vi "Connect Pane.vi"(0 "connect pane":refnum<vi>, 1 "Controls[]":refnum<vi>[](array[refnum]), 11 "error in":errorcluster {"code" format="%.0x"}) -> (3 "Controls[] output":refnum<vi>[](array[refnum]), 4 "connect pane out":refnum<vi>, 15 "error out":errorcluster {"code" format="%.0x"})   [LabVIEW 2018, in "NISAST VI Scripting.lvlib" / "VI.lvlib" / "Connector.lvlib"]
uses:
  Connector.lvlib
  Front Panel/Front Panel.lvlib
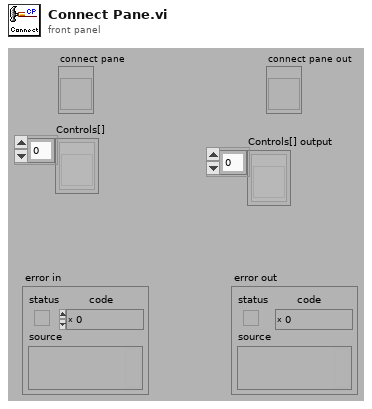
[diagram p1: front panel]
types:
  T1 = typedef "NISAST VI Scripting.lvlib/VI.lvlib/Front Panel.lvlib/Connector Pane Type.ctl" = enum16{"4-2-2-4", "5-2-2-2-5", "Others"}
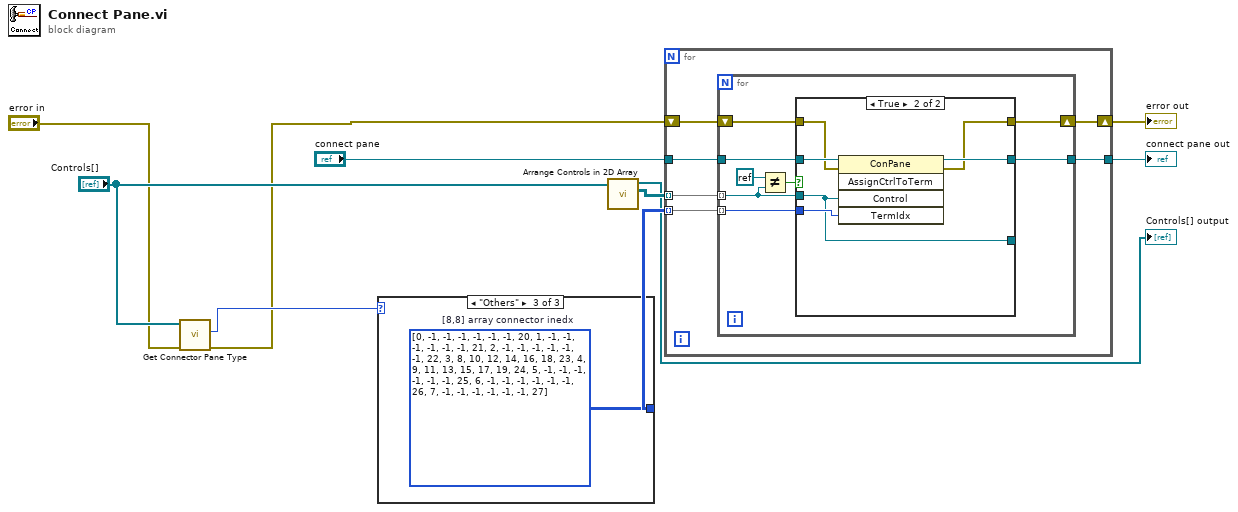
[diagram p0: block diagram]
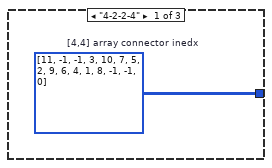
[diagram p2: hidden frame]
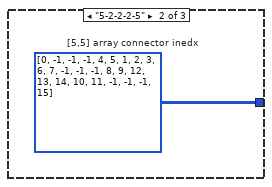
[diagram p3: hidden frame]
diagram:
  n1 = call "Get Connector Pane Type.vi"("error in (no error)"="error in", "Controls[]"="Controls[]") -> ("error out"=w1:errorcluster, "Connector Pane Type"=w3:T1)  [unwired: 7 out]
  n2 = case shown="\"Others\"" w3 {
    tunnel: [w11 w12 w13] -> w6
    frame "4-2-2-4" {
      w11 = i32[][] [[11, -1, -1, 3], [10, 7, 5, 2], [9, 6, 4, 1], [8, -1, -1, 0]]  # [4,4] array connector inedx
    }
    frame "5-2-2-2-5" {
      w12 = i32[][] [[0, -1, -1, -1, 4], [5, 1, 2, 3, 6], [7, -1, -1, -1, 8], [9, 12, 13, 14, 10], [11, -1, -1, -1, 15]]  # [5,5] array connector inedx
    }
    frame "Others" {
      w13 = i32[][] [[0, -1, -1, -1, -1, -1, -1, 20], [1, -1, -1, -1, -1, -1, -1, 21], [2, -1, -1, -1, -1, -1, -1, 22], [3, 8, 10, 12, 14, 16, 18, 23], [4, 9, 11, 13, 15, 17, 19, 24], [5, -1, -1, -1, -1, -1, -1, 25], [6, -1, -1, -1, -1, -1, -1, 26], [7, -1, -1, -1, -1, -1, -1, 27]]  # [8,8] array connector inedx
    }
  }
  n3 = call "Arrange Controls in 2D Array.vi"("Controls[]"="Controls[]") -> ("controls 2D[]"=w7:refnum<vi>[][], "Controls[]"=→"Controls[] output":refnum<vi>[])  [unwired: 1 in, 8 out]
  n4 = for {
    tunnel: w7 -> [w19] mode=indexing
    tunnel: w6 -> [w18] mode=indexing
    tunnel: "connect pane" -> [w17]
    shift-right: [w15] -> w8
    shift-left: w1 -> [w16]
    tunnel: [w14] -> w9
    n5 = for {
      tunnel: w19 -> [w24] mode=indexing
      tunnel: w18 -> [w26] mode=indexing
      tunnel: w17 -> [w25]
      shift-right: [w21] -> w15
      shift-left: w16 -> [w22]
      tunnel: [w20] -> w14
      n6 = Not Equal?(x=refnum<k0> refnum, y=w24) -> (x != y?=w27:bool)
      n7 = case shown="True" w27 {
        tunnel: w24 -> [w28 w32]
        tunnel: w26 -> [_ w34]
        tunnel: w25 -> [w29 w36]
        tunnel: w22 -> [w30 w35]
        tunnel: [w30 w31] -> w21
        tunnel: [w29 w33] -> w20
        tunnel: [w28 w32] -> _
        frame False {
        }
        frame True {
          n8 = invoke class="ConPane" method="AssignCtrlToTerm"(reference=w36, error in=w35, "Control"=w32, "TermIdx"=w34) -> (reference out=w33:refnum<vi>, error out=w31:errorcluster)  [unwired: 1 in, 3 out]
        }
      }
    }
  }
  "error out" <- w8
  "connect pane out" <- w9
